vi "helper_Mono_Setup.vi"(8 "error in":errorcluster) -> (0 "error out":errorcluster, 1 "Module Was Already Running?":bool, 2 "device open for communication?":bool, 3 "Monochromator out":refnum<class "Monochromator.lvclass">)   [LabVIEW 2023, in "horiba.test.lvlib"]
uses:
  horiba.test.lvlib
  Classes/Mono/Monochromator.lvclass
  Classes/DeviceManager/DeviceManager.lvlib
  <userlib>/_OpenG.lib/error/error.llb/openg_error.lvlib
panel:
  # "Connector Pane"
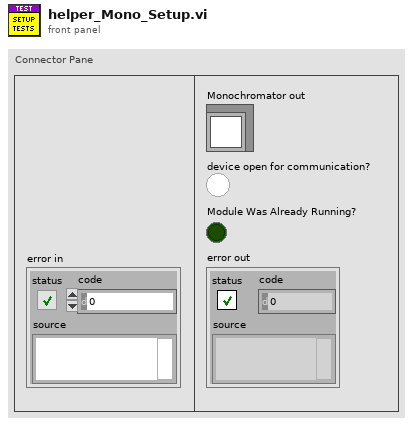
[diagram p1: front panel]
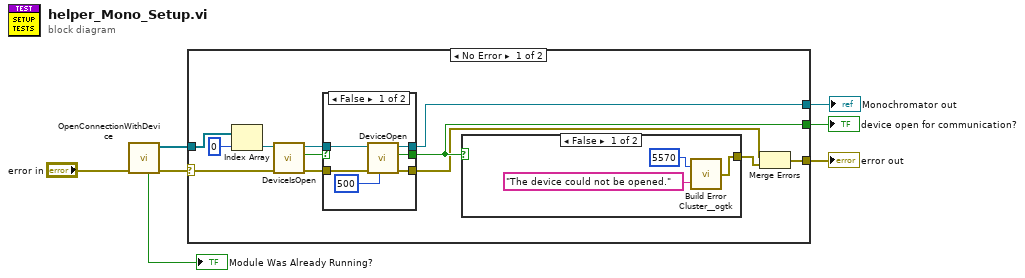
[diagram p0: block diagram]
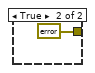
[diagram p3: hidden frame]
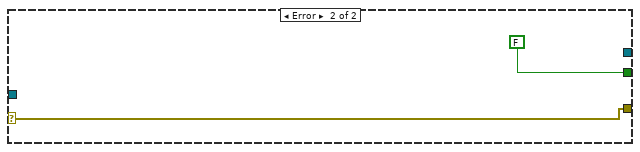
[diagram p4: hidden frame]
diagram:
  n1 = call "OpenConnectionWithDevice.vi"("error in"="error in") -> ("error out"=w4:errorcluster, "Monos"=w3:refnum<class "Monochromator.lvclass">[], "Module Was Already Running?"=→"Module Was Already Running?":bool)  [unwired: 6 in, 2 out]
  n2 = case shown="No Error" w4 {
    selector: w4 -> [w11 w34]
    tunnel: w3 -> [w19 _]
    tunnel: [w17 w34] -> w6
    tunnel: [w15 FALSE ("CCD open for communication?")] -> w5
    tunnel: [w13 _] -> w2
    frame No Error {
      n3 = Index Array(array=w19, index=0) -> (element=w12:refnum<class "Monochromator.lvclass">)
      n4 = call-dynamic "DeviceIsOpen.vi"("error in (no error)"=w11, "Monochromator in"=w12) -> ("error out"=w10:errorcluster, "device is open?"=w9:bool, "Monochromator out"=w8:refnum<class "Monochromator.lvclass">)  [unwired: 6 in, 1 out]
      n5 = case shown="False" w9 {
        selector: w9 -> [_ w26]
        tunnel: [w25 w26] -> w15
        tunnel: [w24 w27] -> w14
        tunnel: [w23 w28] -> w13
        tunnel: w10 -> [w22 w27]
        tunnel: w8 -> [w21 w28]
        frame False {
          n6 = call-dynamic "DeviceOpen.vi"("Delay between send and receive [ms]"=500, "error in (no error)"=w22, "Monochromator in"=w21) -> ("error out"=w24:errorcluster, "device is open?"=w25:bool, "Monochromator out"=w23:refnum<class "Monochromator.lvclass">)  [unwired: 5 in, 1 out]
        }
        frame True {
        }
      }
      n7 = case shown="False" w15 {
        tunnel: [w30 errorcluster {"status"=FALSE, "code"=0, "source"=""} ("error in 2")] -> w16
        frame False {
          n8 = call <userlib>:"Build Error Cluster__ogtk.vi"("String to Prepend to source (\"\")"="The device could not be opened." ("String to Prepend to source (\"\")"), "code"=5570) -> ("error out"=w30:errorcluster)
        }
        frame True {
        }
      }
      n9 = Merge Errors(w14, w16) -> (w17:errorcluster)
    }
    frame Error {
    }
  }
  "error out" <- w6
  "device open for communication?" <- w5
  "Monochromator out" <- w2
